vi "Actor Core.vi"(8 "error in":errorcluster, 11 "Measure Object in":refnum<class "Micron Optics Recorder.lvclass">) -> (0 "error out":errorcluster, 3 "Actor out":refnum<class "Actor.lvclass">)   [LabVIEW 2018, in "Micron Optics Recorder.lvclass"]
doc: "(<B>Filename</B>: Actor Framework.lvlib:Actor.lvclass:Actor Core.vi)\n\nReceives messages to the actor, reacts to them, and initiates any error handling that may shut the actor down.\n\nDescendant classes may override this VI to append parallel tasks for the actor to complete while it handles messages. Overrides use the Call Parent Method node."
uses:
  Micron Optics Recorder.lvclass
  C:/github/LabActor/Template Module/Template Module.lvclass
  C:/github/LabActor/Recorders/Spectrometer/Spectrometer.lvclass
  C:/Program Files/National Instruments/LabVIEW 2018/vi.lib/ActorFramework/Actor/Actor.lvclass
  <vilib>/ActorFramework/Actor/Actor.lvclass
  NHMFL_Core/Libraries/Instruments/Micron Optics/Micron optics configuration.ctl
  Template Module/Template Module.lvclass/Template Module.ctl
  Spectrometer/Spectrometer.lvclass/Spectrometer.ctl
  <vilib>/ActorFramework/Actor/Actor.lvclass/Actor.ctl
  <vilib>/ActorFramework/Message Enqueuer/Message Enqueuer.lvclass/Message Enqueuer.ctl
  Micron Optics Recorder Messages/Plot Spectrum Msg/Plot Spectrum Msg.lvclass/Plot Spectrum Msg.ctl
  Template Module/Read stop event.vi
  Spectrometer/Write Spectrum Graph ref.vi
  <vilib>/ActorFramework/Message Enqueuer/Init from Existing Queue.vi
  <vilib>/ActorFramework/Message Enqueuer/Enqueue.vi
  Micron Optics Recorder Messages/Plot Spectrum Msg/Plot Spectrum Msg.lvclass
  C:/Program Files/National Instruments/LabVIEW 2018/vi.lib/ActorFramework/Message/Message.lvclass
  <vilib>/ActorFramework/Message Priority Queue/Priority Enqueue.vi
  Spectrometer/Spectrometer.lvclass
  <vilib>/ActorFramework/Message Enqueuer/Message Enqueuer.lvclass
panel:
  in  "Channel":u8=1
  in  "Configuration":T1={"Reference channel"=-1, "Detection Setting IDs"=[130, 130], "Address"="192.168.1.55", "Stream and average"=TRUE}
  out "Name":string
  in  "Refresh  specrum":bool
  out "Spectrum Graph":cluster{dbl[], "Spectrum, db":dbl[]}[](graph)
  # "CH1\n.\n.\n.\n.\n.\nCH4"
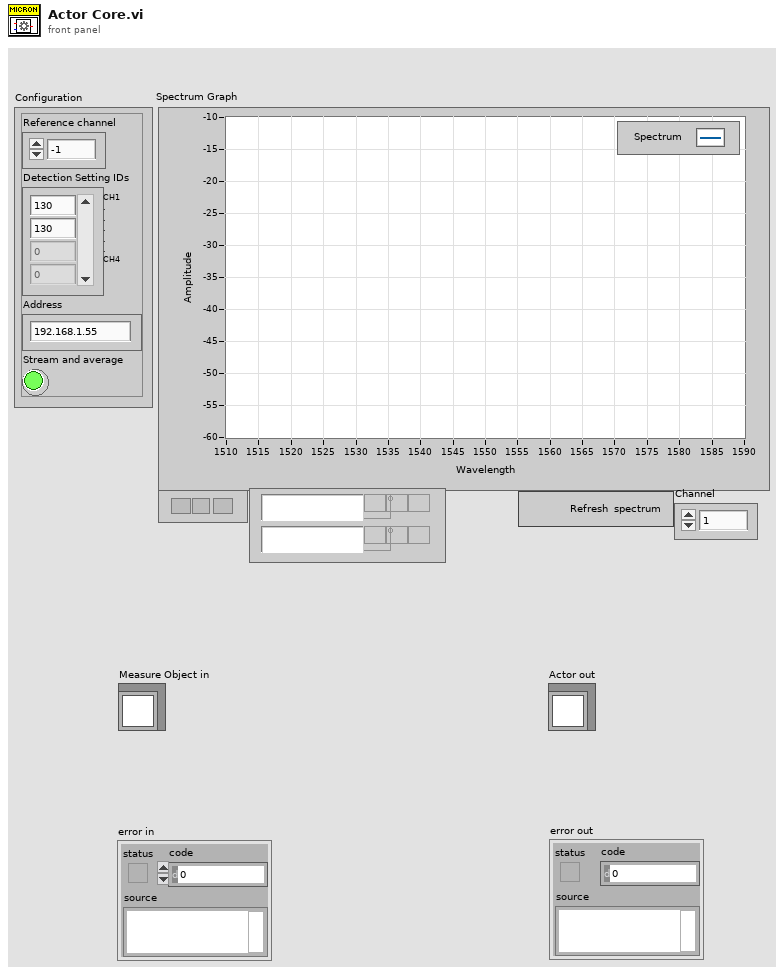
[diagram p1: front panel]
types:
  T1 = typedef "Micron optics configuration.ctl" = cluster{"Reference channel":i32, "Detection Setting IDs":u8[], "Address":string, "Stream and average":bool}
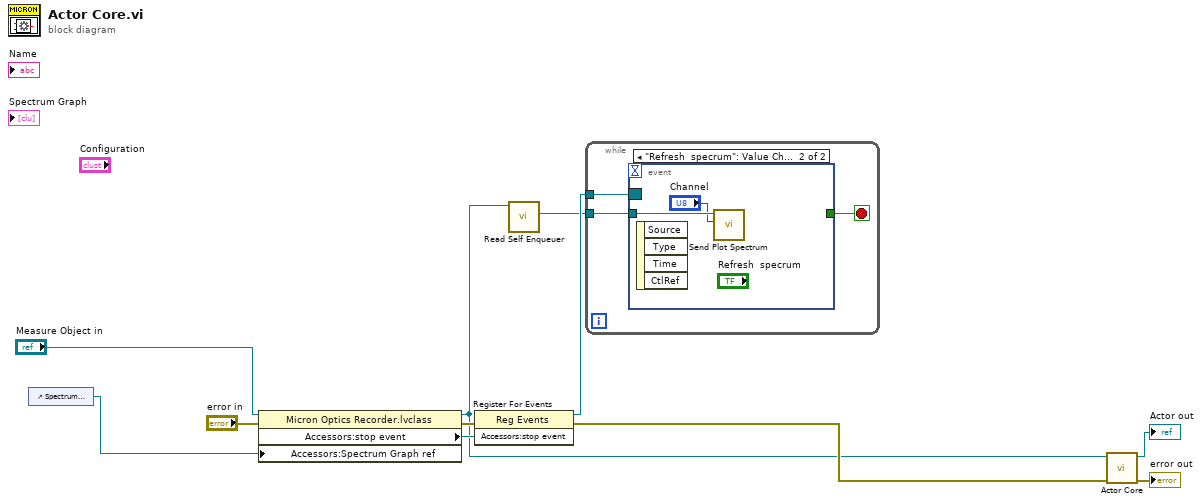
[diagram p0: block diagram]
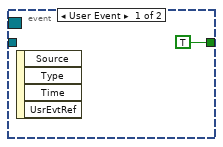
[diagram p2: hidden frame]
diagram:
  n1 = control-ref of="Spectrum Graph"() -> (w1:refnum<vi>)
  n2 = property class="Micron Optics Recorder.lvclass"(reference="Measure Object in", error in="error in", "Accessors:Spectrum Graph ref"=w1) -> (reference out=w4:refnum<class "Micron Optics Recorder.lvclass">, error out=w8:errorcluster, "Accessors:stop event"=w9:refnum<user-event>)
  n3 = register-events(error in=w8, w9) -> (reference out=w3:refnum<event-registration>, error out=w5:errorcluster)  [unwired: 1 in]
  n4 = call <vilib>:"Read Self Enqueuer.vi"("Actor"=w4) -> ("Self Enqueuer"=w2:refnum<class "Message Enqueuer.lvclass">)  [unwired: 10 in]
  n5 = while {
    tunnel: w3 -> [w14]
    tunnel: w2 -> [w12]
    stop <- w13 stop-if-true
    n6 = event shown="[1] \"Refresh  specrum\": Value Change" {
      selector: w14 -> [_ _]
      dyn-events: _ -> [_ _]
      timeout: _ -> [_ _]
      tunnel: [TRUE _] -> w13
      tunnel: w12 -> [_ w17]
      event User Event {
        n7 = event-data() -> ()  [unwired: 1 in, 4 out]
      }
      event "Refresh  specrum": Value Change {
        n8 = event-data() -> ()  [unwired: 1 in, 4 out]
        n9 = call "Send Plot Spectrum.vi"("Channel"="Channel", "Message Enqueuer"=w17) -> ()  [unwired: 8 in, 2 out]
      }
    }
  }
  n10 = call-parent "Actor Core.vi"("error in"=w5, "Measure Object in"=w4) -> ("error out"=→"error out":errorcluster, "Actor out"=→"Actor out":refnum<class "Actor.lvclass">)  [unwired: 8 in]
